vi "WFParameters.vi"(6 "Baseline (V)":dbl, 8 "Dur (s)":dbl=0.25, 9 "Ramp (s)":dbl=0.005, 10 "Amp (V)":dbl=1.0, 11 "Fs (Hz)":dbl=100000.0 min=1.0) -> (3 "WFParameters":T1={"Fs (Hz)"=100000.0, "Amp (V)"=1.0, "Ramp (s)"=0.005, "Dur (s)"=0.25, "Baseline (V)"=0.0} {"Dur (s)" min=0.0 format="%#_4g"; "Ramp (s)" min=0.0; "Fs (Hz)" min=0.0})   [LabVIEW 2013]
uses:
  WFParameters.ctl
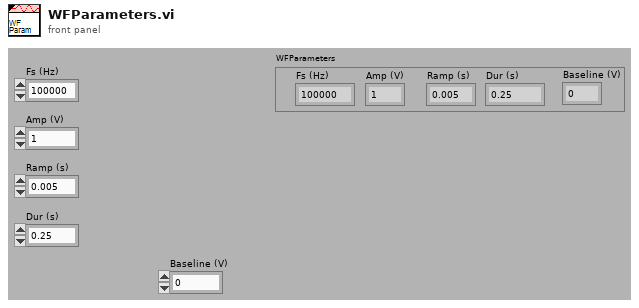
[diagram p1: front panel]
types:
  T1 = typedef "WFParameters.ctl" = cluster{"Fs (Hz)":dbl, "Amp (V)":dbl, "Ramp (s)":dbl, "Dur (s)":dbl, "Baseline (V)":dbl}
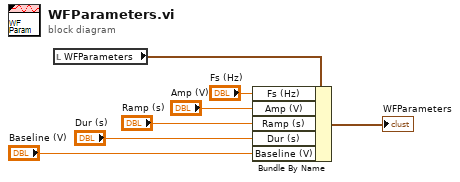
[diagram p0: block diagram]
diagram:
  n1 = local read "WFParameters"() -> (w6:T1)
  n2 = Bundle By Name(cluster=w6, "Fs (Hz)"="Fs (Hz)", "Amp (V)"="Amp (V)", "Ramp (s)"="Ramp (s)", "Dur (s)"="Dur (s)", "Baseline (V)"="Baseline (V)") -> (→"WFParameters":T1)
